vi "Fetch (Math).vi"(0 "VISA resource name":refnum<visa-resource-name>, 5 "Timeout (10000 ms)":i32=10000 format="%#.6g", 11 "error in (no error)":errorcluster) -> (4 "VISA resource name out":refnum<visa-resource-name>, 6 "Math Results":sgl[](array[numeric]), 15 "error out":errorcluster)   [LabVIEW 2015, in "VIPM2.lvlib" / "Keithley 24XX.lvlib"]
doc: "Fetches the data from the math buffer.\n\n<B>Note</B> Use this VI only with other low-level VIs. The high-level VIs automatically incorporate this functionality. This VI does not check the instrument status. If you want to check the instrument status, call the Error Query VI at the conclusion of the sequence."
uses:
  Keithley 24XX.lvlib
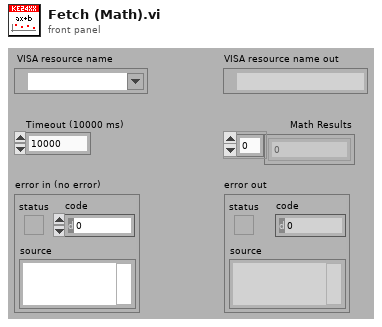
[diagram p1: front panel]
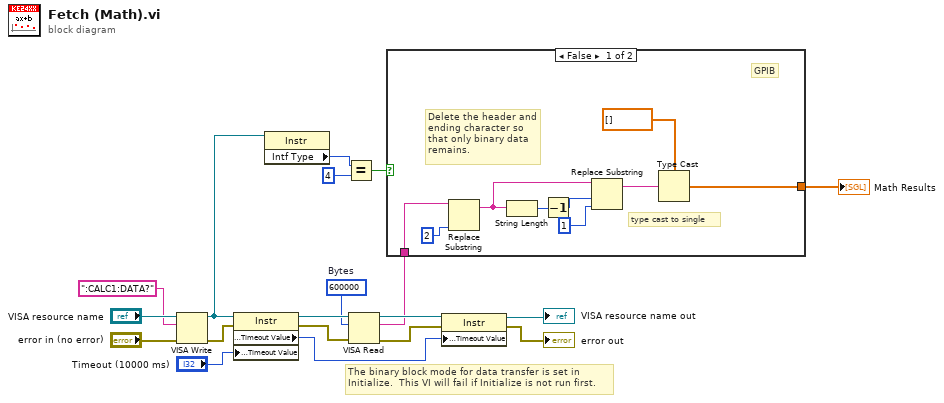
[diagram p0: block diagram]
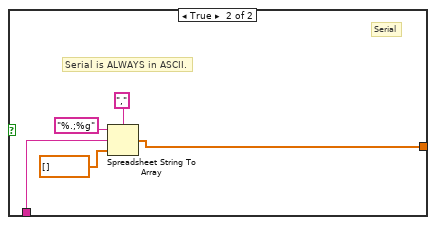
[diagram p2: hidden frame]
diagram:
  w8 = u32 600000  # Bytes
  # "The binary block mode for data transfer is set in Initialize.  This VI will fail if Initialize is not run first."
  n1 = VISA Write(VISA resource name="VISA resource name", write buffer=":CALC1:DATA?", error in (no error)="error in (no error)") -> (VISA resource name out=w1:refnum<visa-resource-name>, error out=w17:errorcluster)  [unwired: 1 out]
  n2 = property class="Instr"(reference=w1, error in=w17, "General Settings:Timeout Value"="Timeout (10000 ms)") -> (reference out=w16:refnum<visa-resource-name>, error out=w15:errorcluster, "General Settings:Timeout Value"=w11:u32)
  n3 = property class="Instr"(reference=w1) -> ("Intf Type"=w4:u16)  [unwired: 1 in, 2 out]
  n4 = Equal?(x=w4, y=u16 4) -> (x = y?=w2:bool)
  n5 = VISA Read(VISA resource name=w16, byte count=w8, error in (no error)=w15) -> (VISA resource name out=w13:refnum<visa-resource-name>, read buffer=w5:string, error out=w12:errorcluster)  [unwired: 1 out]
  n6 = case shown="False" w2 {
    tunnel: w5 -> [w28 w33]
    tunnel: [w20 w29] -> w6
    frame False {
      # "Delete the header and ending character so that only binary data remains."
      # "GPIB"
      # "type cast to single"
      n7 = Replace Substring(2:2 ("length (len. of substring)"), 5:w28) -> (1:w26:string)  [unwired: 2 in, 1 out]
      n8 = String Length(string=w26) -> (length=w25:i32)
      n9 = Decrement(x=w25) -> (x-1=w24:i32)
      n10 = Replace Substring(2:1 ("length (len. of substring)"), 3:w24, 5:w26) -> (1:w22:string)  [unwired: 1 in, 1 out]
      n11 = Type Cast(type=sgl[] [], x=w22) -> (*(type *) &x=w20:sgl[])
    }
    frame True {
      # "Serial is ALWAYS in ASCII."
      # "Serial"
      n12 = Spreadsheet String To Array(delimiter (Tab)=",", format string="%.;%g", spreadsheet string=w33, array type (2D Dbl)=sgl[] []) -> (array=w29:sgl[])
    }
  }
  "Math Results" <- w6
  n13 = property class="Instr"(reference=w13, error in=w12, "General Settings:Timeout Value"=w11) -> (reference out=→"VISA resource name out":refnum<visa-resource-name>, error out=→"error out":errorcluster)
